vi "IND560 Seperate String Numbers.vi"(11 "read buffer":string) -> (2 "Gross Weight":string, 3 "Net Weight":string)   [LabVIEW 2019]
uses:
  <vilib>/Utility/error.llb/whitespace.ctl
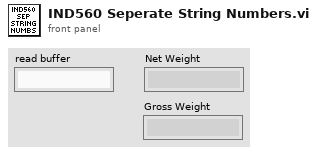
[diagram p1: front panel]
types:
  T1 = typedef "whitespace.ctl" = u16
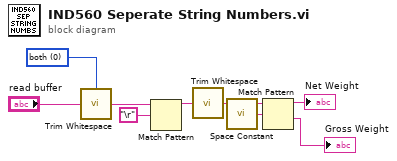
[diagram p0: block diagram]
diagram:
  w6 = T1 0 items=["both", "start of string", "end of string"] ("location (both)")
  n1 = call <vilib>:"Trim Whitespace.vi"("string"="read buffer", "location (both)"=w6) -> ("trimmed string"=w8:string)
  n2 = Match Pattern(string=w8, regular expression="\r") -> (before substring=w4:string)  [unwired: 1 in, 3 out]
  n3 = call <vilib>:"Trim Whitespace.vi"("string"=w4) -> ("trimmed string"=w5:string)  [unwired: 1 in]
  n4 = call <vilib>:"Space Constant.vi"() -> ("String"=w3:string)
  n5 = Match Pattern(string=w5, regular expression=w3) -> (before substring=→"Net Weight":string, after substring=→"Gross Weight":string)  [unwired: 1 in, 2 out]
